vi "Search HPS Network.vi"(0 "reference in":refnum<class "HPS-17000-PowerModule.lvclass">, 11 "Error In":errorcluster) -> (4 "reference out":refnum<class "HPS-17000-PowerModule.lvclass">, 15 "Error Out":errorcluster)   [LabVIEW 2023]
uses:
  HPS-17000-PowerModule.lvclass
  HPS-17000-PowerModule.lvclass/HPS-17000-PowerModule.ctl
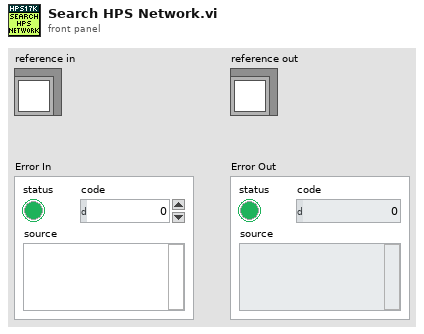
[diagram p1: front panel]
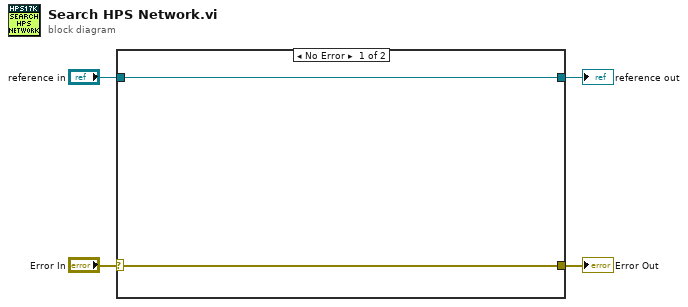
[diagram p0: block diagram]
diagram:
  n1 = case shown="No Error" "Error In" {
    selector: "Error In" -> [w5 w8]
    tunnel: [w5 w8] -> w3
    tunnel: [w6 w7] -> w1
    tunnel: "reference in" -> [w6 w7]
    frame No Error {
    }
    frame Error {
    }
  }
  "Error Out" <- w3
  "reference out" <- w1
